vi "CS-4 Initialize.vi"(8 "error in (no error)":errorcluster, 9 "Reset (T: Reset)":bool=TRUE, 10 "ID Query (T: Check)":bool=TRUE, 11 "VISA session (for class)":refnum<visa-resource-name>) -> (0 "error out":errorcluster, 3 "VISA session":refnum<visa-resource-name>)   [LabVIEW 2016]
doc: "This VI passes the addressing information in the instrument decriptor to the Instr Open VI and returns the instrument ID. You can optionally reset the instrument by setting the front panel reset control. You must run this VI before using any of the instrument driver VIs for this instrument."
panel:
  # "Check\nDon't Check"
  # "Reset\nDon't Reset"
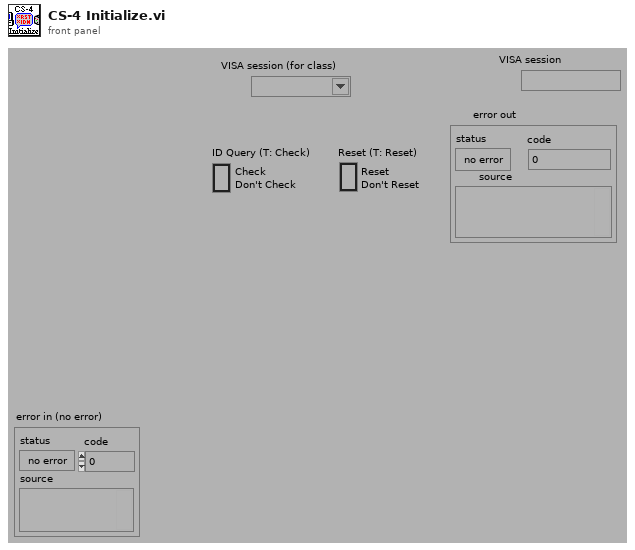
[diagram p1: front panel]
types:
  T1 = cluster{"status":bool, "code":i32, "VI name":string}
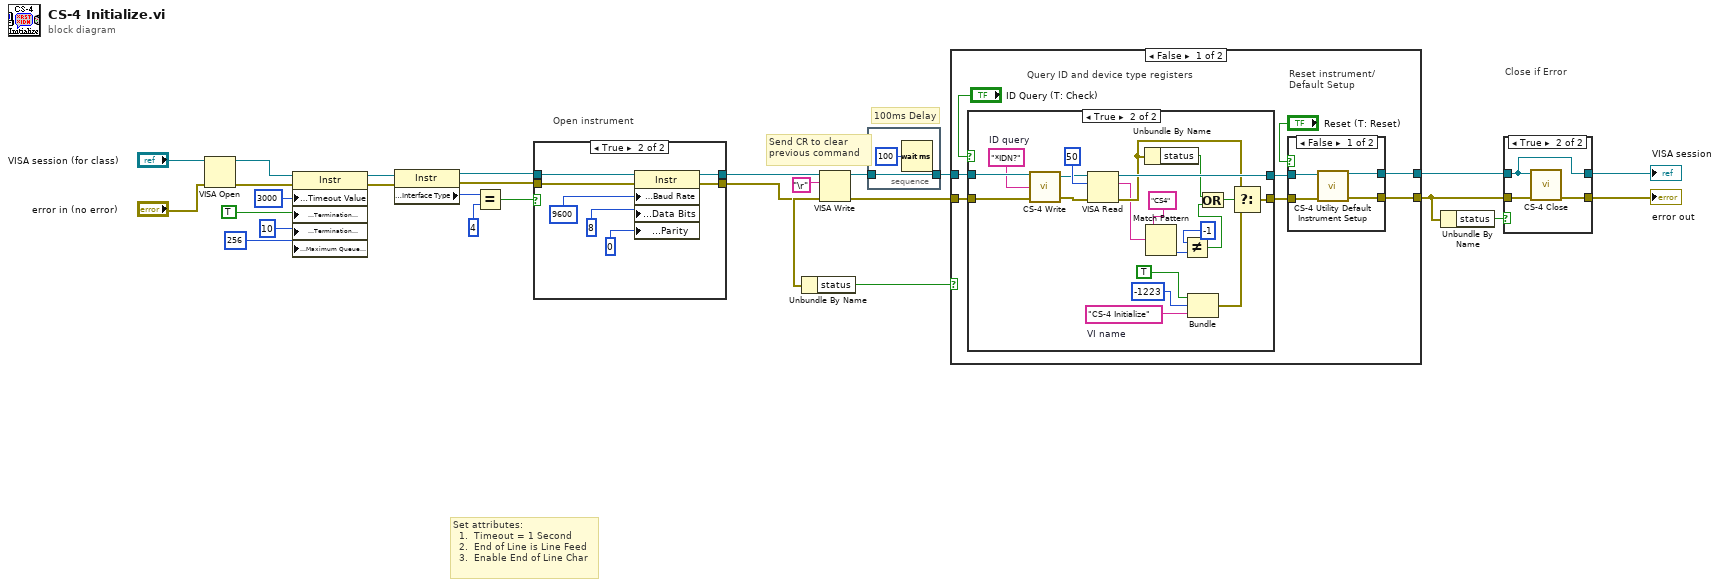
[diagram p0: block diagram]
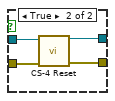
[diagram p5: hidden frame]
diagram:
  # "100ms Delay"
  # "Send CR to clear\nprevious command"
  # "Close if Error"
  # "Set attributes:\n  1.  Timeout = 1 Second\n  2.  End of Line is Line Feed\n  3.  Enable End of Line Char"
  # "Open instrument"
  n1 = VISA Open(error in (no error)="error in (no error)", VISA resource name="VISA session (for class)") -> (VISA resource name=w2:refnum<visa-resource-name>, error out=w4:errorcluster)  [unwired: 3 in]
  n2 = property class="Instr"(reference=w2, error in=w4, "General Settings:Timeout Value"=u32 3000 ("Tmo Value"), "Message Based Settings:Termination Character Enable"=TRUE ("TermChar En"), "Message Based Settings:Termination Character"=u8 10 ("TermChar"), "General Settings:Maximum Queue Length"=u32 256 ("Max Queue Len")) -> (reference out=w9:refnum<visa-resource-name>, error out=w7:errorcluster)
  n3 = property class="Instr"(reference=w9, error in=w7) -> (reference out=w8:refnum<visa-resource-name>, error out=w6:errorcluster, "Interface Information:Interface Type"=w5:u16)
  n4 = Equal?(x=w5, y=u16 4) -> (x = y?=w10:bool)
  n5 = case shown="True" w10 {
    tunnel: [w29 w32] -> w1
    tunnel: w8 -> [w29 w31]
    tunnel: w6 -> [w28 w30]
    tunnel: [w28 w33] -> w3
    frame False {
    }
    frame True {
      n6 = property class="Instr"(reference=w31, error in=w30, "Serial Settings:Baud Rate"=u32 9600 ("ASRL Baud"), "Serial Settings:Data Bits"=u32 8 ("Tmo Value"), "Serial Settings:Parity"=u16 0 ("ASRL Parity")) -> (reference out=w32:refnum<visa-resource-name>, error out=w33:errorcluster)
    }
  }
  n7 = VISA Write(VISA resource name=w1, write buffer="\r", error in (no error)=w3) -> (VISA resource name out=w17:refnum<visa-resource-name>, error out=w18:errorcluster)  [unwired: 1 out]
  n8 = Unbundle By Name(w18) -> ("status"=w25:bool)
  n9 = stacked-sequence {
    tunnel: w17 -> [w37]
    tunnel: [w37] -> w16
    frame #0 {
      n10 = Wait (ms)(milliseconds to wait=u32 100) -> ()  [unwired: 1 out]
    }
  }
  n11 = case shown="False" w25 {
    tunnel: w18 -> [w46 w77]
    tunnel: w16 -> [w45 w78]
    tunnel: [w40 w77] -> w21
    tunnel: [w39 w78] -> w24
    frame False {
      # "Reset instrument/\nDefault Setup"
      # "Query ID and device type registers"
      n12 = case shown="True" "ID Query (T: Check)" {
        tunnel: [w47 w68] -> w42
        tunnel: [w48 w65] -> w41
        tunnel: w45 -> [w48 w66]
        tunnel: w46 -> [w47 w67]
        frame False {
        }
        frame True {
          w61 = "*IDN?"  # ID query
          w50 = "CS-4 Initialize"  # VI name
          n13 = call "CS-4 Write.vi"("error in (no error)"=w67, "write buffer (\"\")"=w61, "VISA session"=w66) -> ("error out"=w54:errorcluster, "dup VISA session"=w52:refnum<visa-resource-name>)  [unwired: 1 out]
          n14 = VISA Read(VISA resource name=w52, byte count=u32 50, error in (no error)=w54) -> (VISA resource name out=w65:refnum<visa-resource-name>, read buffer=w49:string, error out=w53:errorcluster)  [unwired: 1 out]
          n15 = Unbundle By Name(w53) -> ("status"=w56:bool)
          n16 = Match Pattern(string=w49, regular expression="CS4") -> (offset past match=w59:i32)  [unwired: 1 in, 3 out]
          n17 = Not Equal?(x=-1, y=w59) -> (x != y?=w51:bool)
          n18 = Bundle(TRUE, -1223, "VI name"=w50) -> (w62:cluster{bool, i32, "VI name":string})  [unwired: 1 in]
          n19 = Or(x=w56, y=w51) -> (x .or. y?=w55:bool)
          n20 = Select(t=w53, s=w55, f=w62) -> (s? t:f=w68:T1)
        }
      }
      n21 = case shown="False" "Reset (T: Reset)" {
        tunnel: w42 -> [w71 w73]
        tunnel: [w70 w76] -> w40
        tunnel: w41 -> [w72 w74]
        tunnel: [w69 w75] -> w39
        frame False {
          n22 = call "CS-4 Utility Default Instrument Setup.vi"("error in (no error)"=w71, "VISA session"=w72) -> ("error out"=w70:errorcluster, "dup VISA session"=w69:refnum<visa-resource-name>)  [unwired: 8 in]
        }
        frame True {
          n23 = call "CS-4 Reset.vi"("error in (no error)"=w73, "VISA session"=w74) -> ("error out"=w76:errorcluster, "dup VISA session"=w75:refnum<visa-resource-name>)  [unwired: 8 in]
        }
      }
    }
    frame True {
    }
  }
  n24 = Unbundle By Name(w21) -> ("status"=w20:bool)
  n25 = case shown="True" w20 {
    tunnel: [w80 w81] -> w23
    tunnel: [w79 w83] -> w22
    tunnel: w21 -> [w79 w82]
    tunnel: w24 -> [w80 w81]
    frame False {
    }
    frame True {
      n26 = call "CS-4 Close.vi"("error in (no error)"=w82, "VISA session"=w81) -> ("error out"=w83:errorcluster)  [unwired: 9 in]
    }
  }
  "VISA session" <- w23
  "error out" <- w22
